vi "Demo_DB Path.vi"(8 "error in":errorcluster) -> (0 "error out":errorcluster, 3 "DB Path":path)   [LabVIEW 2017]
panel:
  # "DESKTOP-D1JM1FD\\SQLEXPRESS"
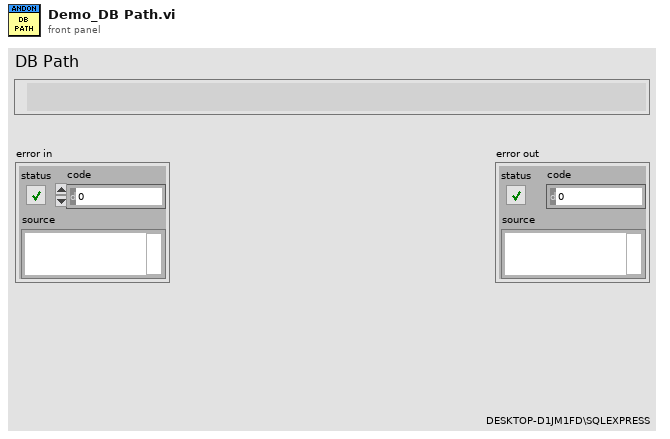
[diagram p1: front panel]
types:
  T1 = enum32{"invalid app kind", "Development System", "Run Time System", "Student Edition", "Embedded LabVIEW", "Evaluation", "Custom"}
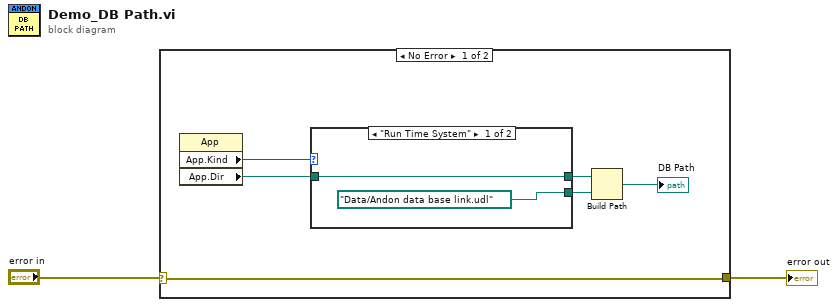
[diagram p0: block diagram]
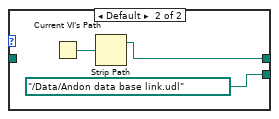
[diagram p2: hidden frame]
diagram:
  n1 = case shown="No Error" "error in" {
    selector: "error in" -> [w4 w14]
    tunnel: [w4 w14] -> w1
    frame No Error {
      n2 = property class="App"() -> ("App.Kind"=w8:T1, "App.Dir"=w7:path)  [unwired: 2 in, 2 out]
      n3 = case shown="\"Run Time System\"" w8 {
        tunnel: w7 -> [w10 _]
        tunnel: [path "Data/Andon data base link.udl" ("path") path "../Data/Andon data base link.udl" ("path")] -> w6
        tunnel: [w10 w11] -> w5
        frame "Run Time System" {
        }
        frame Default {
          n4 = Current VI's Path() -> (path=w12:path)
          n5 = Strip Path(path=w12) -> (stripped path=w11:path)  [unwired: 1 out]
        }
      }
      n6 = Build Path(base path=w5, name or relative path=w6) -> (appended path=→"DB Path":path)
    }
    frame Error {
    }
  }
  "error out" <- w1
